vi "PXI-Zero 16-bit Outputs (by device).vi"(8 "error in (no error)":errorcluster, 11 "DevNames":tag[](array[tag])) -> (0 "error out":errorcluster)   [LabVIEW 2020]
uses:
  <vilib>/DAQmx/write.llb/DAQmx Write (Analog 2D DBL NChan NSamp).vi
  <vilib>/DAQmx/create/channels.llb/DAQmx Create Channel (AO-Voltage-Basic).vi
  <vilib>/DAQmx/configure/timing.llb/DAQmx Timing (Sample Clock).vi
  <vilib>/DAQmx/miscellaneous.llb/DAQmx Fill In Error Info.vi
  <resource>/objmgr/daqmx.rc
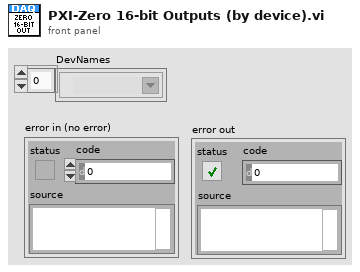
[diagram p1: front panel]
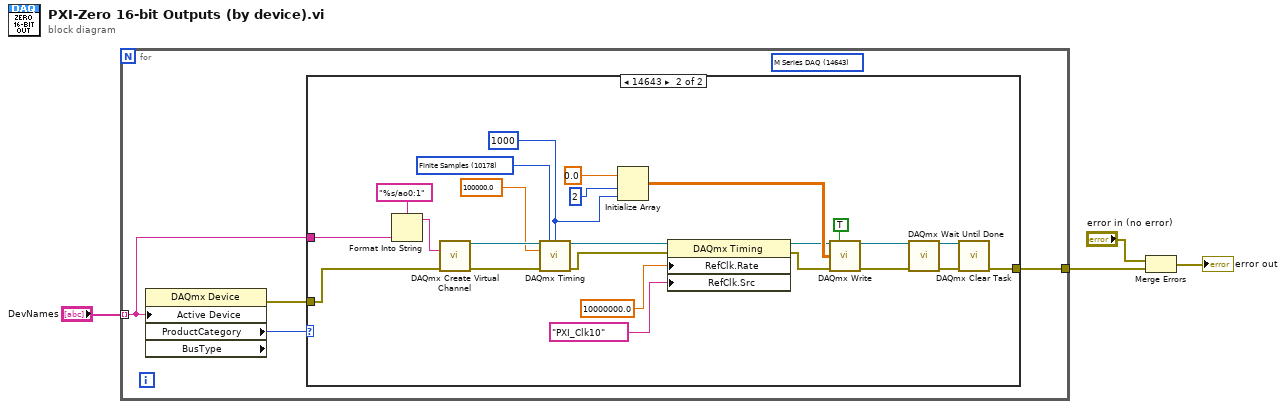
[diagram p0: block diagram]
diagram:
  n1 = for {
    tunnel: "DevNames" -> [w6] mode=indexing
    tunnel: [w7] -> w4
    (unwired) 14643 items=["M Series DAQ"=14643, "X Series DAQ"=15858, "E Series DAQ"=14642, "S Series DAQ"=14644, "B Series DAQ"=14662, "SC Series DAQ"=14645, "USB DAQ"=14646, "AO Series"=14647, "Digital I/O"=14648, "TIO Series"=14661, "Dynamic Signal Acquisition"=14649, "Switches"=14650, "CompactDAQ Chassis"=14658, "C Series Module"=14659, "SCXI Module"=14660, "SCC Connector Block"=14704, "SCC Module"=14705, "NI ELVIS"=14755, "Network DAQ"=14829, "SC Express"=15886, "Unknown"=12588] ("ProductCategory")
    n2 = property class="DAQmx Device" props=["Active Device", "ProductCategory", "BusType"]("Active Device"=w6) -> (error out=w8:errorcluster, "ProductCategory"=w5:i32)  [unwired: 2 in, 2 out]
    n3 = case shown="14643" w5 {
      tunnel: w8 -> [_ w30]
      tunnel: [_ w32] -> w7
      tunnel: w6 -> [_ w31]
      frame 0, Default {
      }
      frame 14643 {
        w17 = 1000 ("samples per channel")
        w24 = 10178 items=["Finite Samples"=10178, "Continuous Samples"=10123, "Hardware Timed Single Point"=12522] ("sample mode")
        n4 = Format Into String(format string="%s/ao0:1" ("physical channels"), w31) -> (resulting string=w16:string)  [unwired: 2 in, 1 out]
        n5 = call-poly <vilib>:"DAQmx Create Virtual Channel.vi"("physical channels"=w16, "error in"=w30) -> ("task out"=w26:refnum<k21>, "error out"=w25:errorcluster)  [unwired: 12 in]
        n6 = call-poly <vilib>:"DAQmx Timing.vi"("task/channels in"=w26, "sample mode"=w24, "samples per channel"=w17, "rate"=100000.0, "error in"=w25) -> ("task out"=w12:refnum<k21>, "error out"=w9:errorcluster)  [unwired: 9 in]
        n7 = Initialize Array(0.0 ("element"), 2 ("dimension size"), w17) -> (w20:dbl[][])
        n8 = property class="DAQmx Timing"(reference=w12, error in=w9, "RefClk.Rate"=10000000.0, "RefClk.Src"=tag "PXI_Clk10") -> (reference out=w11:refnum<k21>, error out=w10:errorcluster)
        n9 = call-poly <vilib>:"DAQmx Write.vi"("task/channels in"=w11, "auto start"=TRUE, "data"=w20, "error in"=w10) -> ("task out"=w22:refnum<k21>, "error out"=w21:errorcluster)  [unwired: 9 in, 1 out]
        n10 = call <vilib>:"DAQmx Wait Until Done.vi"("task/channels in"=w22, "error in"=w21) -> ("task out"=w28:refnum<k21>, "error out"=w27:errorcluster)  [unwired: 12 in]
        n11 = call <vilib>:"DAQmx Clear Task.vi"("task in"=w28, "error in"=w27) -> ("error out"=w32:errorcluster)  [unwired: 13 in]
      }
    }
  }
  n12 = Merge Errors("error in (no error)", w4) -> (→"error out":errorcluster)
